vi "Bridge1_Main.vi"(5 "error in (no error)":errorcluster) -> (19 "error out":errorcluster)   [LabVIEW 2020]
doc: "</summary>"
uses:
  CustomersData_class/CustomersData.lvclass
  C:/Projects/DesignPatterns_Trunk/Bridge/DataObject_class/DataObject.lvclass
  Customers_class/Customers.lvclass
panel:
  out "String":string
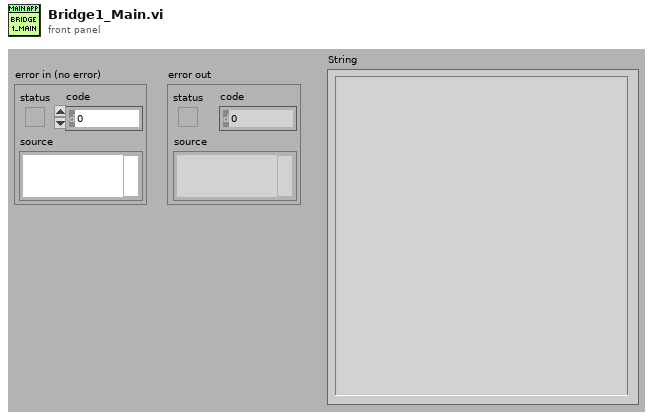
[diagram p1: front panel]
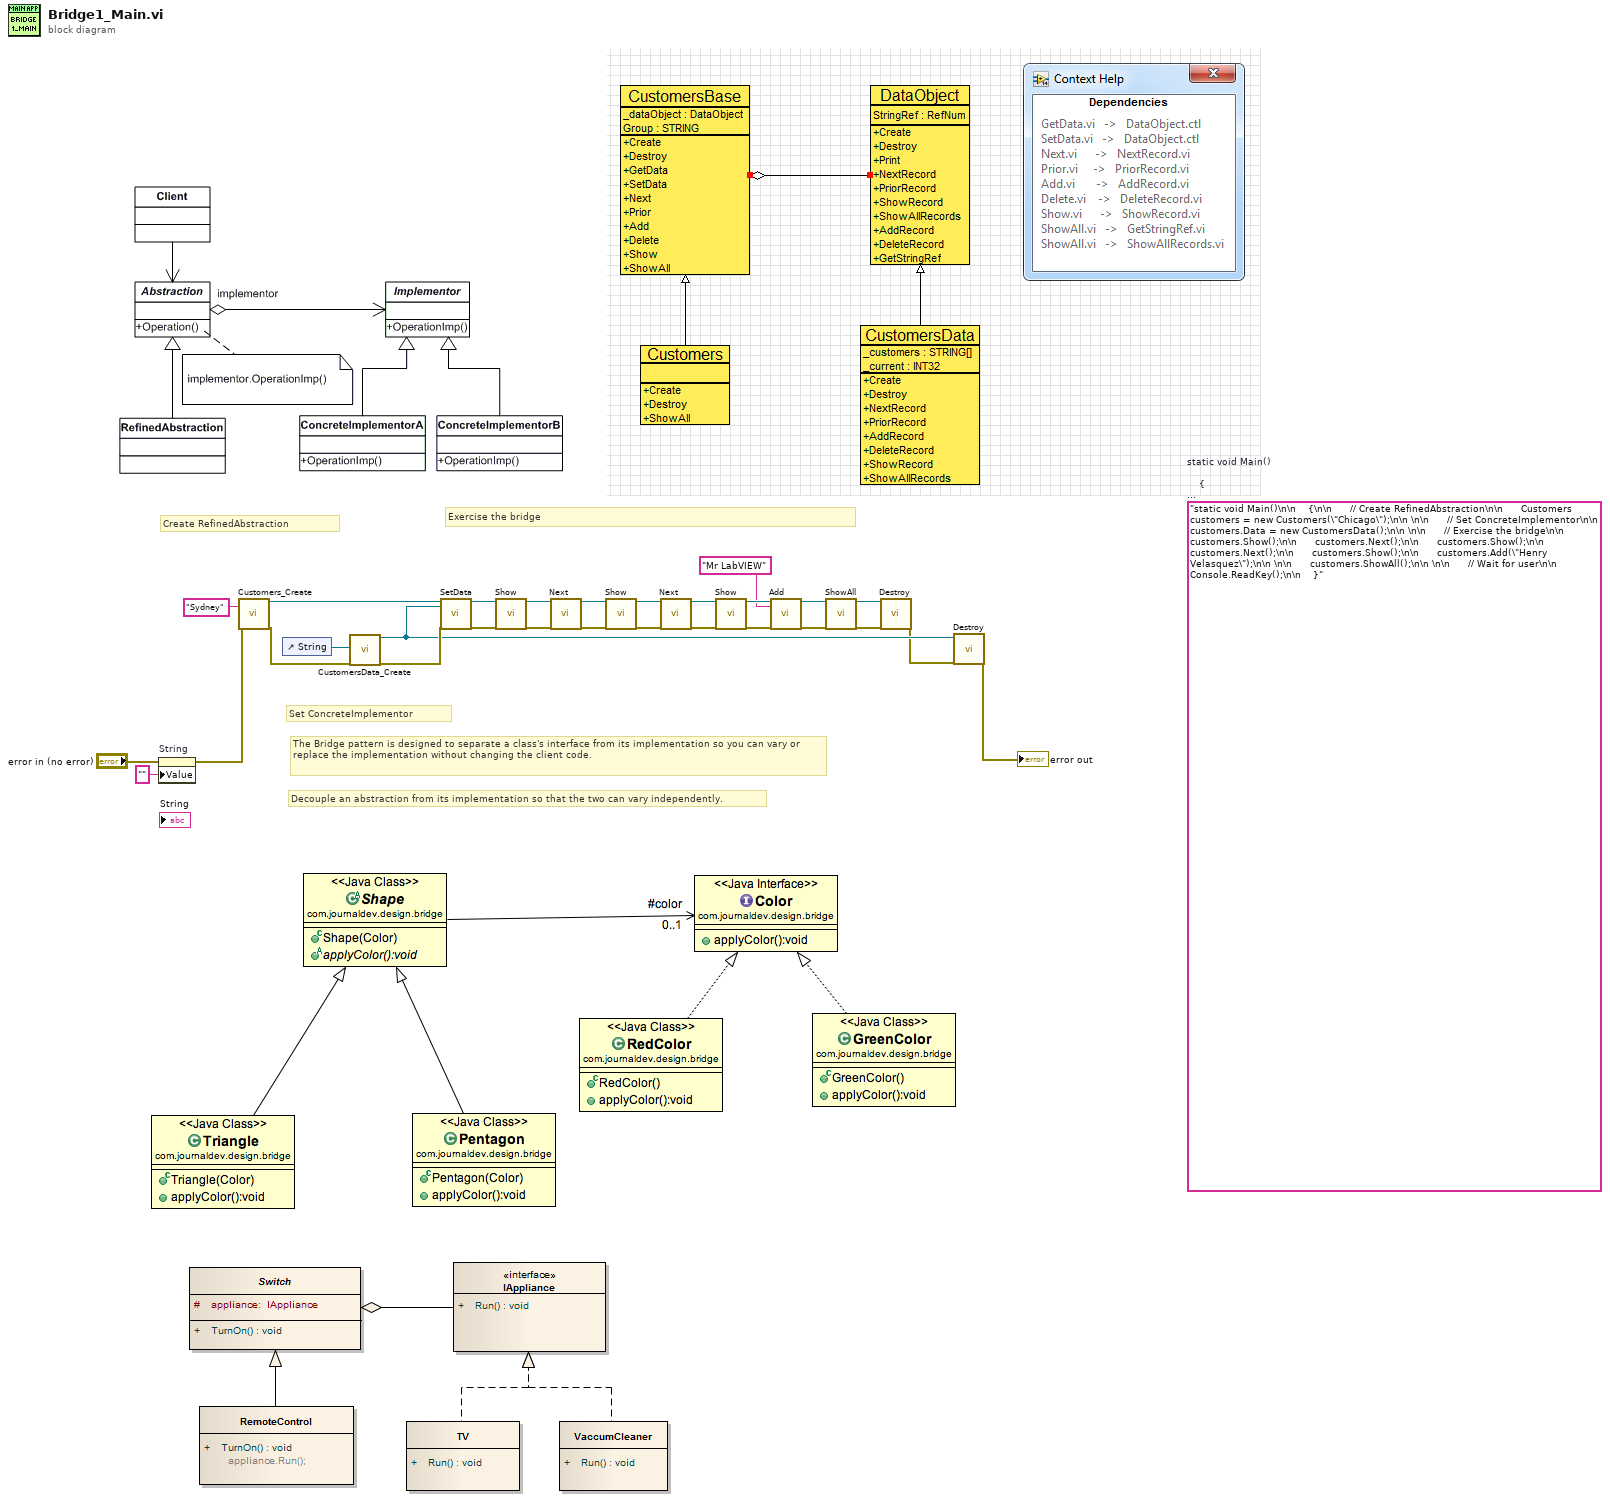
[diagram p0: block diagram]
diagram:
  (unwired) "static void Main()\n\n    {\n\n      // Create RefinedAbstraction\n\n      Customers customers = new Customers(\"Chicago\");\n\n \n\n      // Set ConcreteImplementor\n\n      customers.Data = new CustomersData();\n\n \n\n      // Exercise the bridge\n\n      customers.Show();\n\n      customers.Next();\n\n      customers.Show();\n\n      customers.Next();\n\n      customers.Show();\n\n      customers.Add(\"Henry Velasquez\");\n\n \n\n      customers.ShowAll();\n\n \n\n      // Wait for user\n\n      Console.ReadKey();\n\n    }"  # static void Main()      {        // Create RefinedAbstraction        Customers customers = new Customers("Chicago");           // Set ConcreteImplementor        customers.Data = new CustomersData();           // Exercise the bridge        customers.Show();        customers.Next();        customers.Show();        customers.Next();        customers.Show();        customers.Add("Henry Velasquez");           customers.ShowAll();           // Wait for user        Console.ReadKey();      }
  # "Decouple an abstraction from its implementation so that the two can vary independently."
  # "The Bridge pattern is designed to separate a class's interface from its implementation so you can vary or replace the implementation without changing the client code."
  # "Exercise the bridge"
  # "Set ConcreteImplementor"
  # "Create RefinedAbstraction"
  n1 = property on="String" class="Str"(error in="error in (no error)", "Value"="" ("String")) -> (error out=w2:errorcluster)  [unwired: 1 in, 1 out]
  n2 = call "Customers_Create.vi"("Group"="Sydney", "error in (no error)"=w2) -> ("reference out"=w27:refnum<class "Customers.lvclass">, "error out"=w26:errorcluster)  [unwired: 16 in]
  n3 = control-ref of="String"() -> (w4:refnum<vi>)
  n4 = call "CustomersData_Create.vi"("StringRef"=w4, "error in (no error)"=w26) -> ("reference out"=w7:refnum<class "CustomersData.lvclass">, "error out"=w25:errorcluster)  [unwired: 16 in]
  n5 = call-dynamic "SetData.vi"("reference in"=w27, "Data"=w7, "error in (no error)"=w25) -> ("reference out"=w23:refnum<class "Customers.lvclass">, "error out"=w24:errorcluster)  [unwired: 15 in]
  n6 = call-dynamic "Show.vi"("reference in"=w23, "error in (no error)"=w24) -> ("reference out"=w21:refnum<class "Customers.lvclass">, "error out"=w22:errorcluster)  [unwired: 16 in]
  n7 = call-dynamic "Next.vi"("reference in"=w21, "error in (no error)"=w22) -> ("reference out"=w18:refnum<class "Customers.lvclass">, "error out"=w17:errorcluster)  [unwired: 16 in]
  n8 = call-dynamic "Show.vi"("reference in"=w18, "error in (no error)"=w17) -> ("reference out"=w20:refnum<class "Customers.lvclass">, "error out"=w19:errorcluster)  [unwired: 16 in]
  n9 = call-dynamic "Next.vi"("reference in"=w20, "error in (no error)"=w19) -> ("reference out"=w16:refnum<class "Customers.lvclass">, "error out"=w15:errorcluster)  [unwired: 16 in]
  n10 = call-dynamic "Show.vi"("reference in"=w16, "error in (no error)"=w15) -> ("reference out"=w13:refnum<class "Customers.lvclass">, "error out"=w14:errorcluster)  [unwired: 16 in]
  n11 = call-dynamic "Add.vi"("reference in"=w13, "Customer"="Mr LabVIEW" ("Group"), "error in (no error)"=w14) -> ("reference out"=w11:refnum<class "Customers.lvclass">, "error out"=w10:errorcluster)  [unwired: 15 in]
  n12 = call-dynamic "ShowAll.vi"("reference in"=w11, "error in (no error)"=w10) -> ("reference out"=w8:refnum<class "Customers.lvclass">, "error out"=w9:errorcluster)  [unwired: 16 in]
  n13 = call-dynamic "Destroy.vi"("reference in"=w8, "error in (no error)"=w9) -> ("error out"=w6:errorcluster)  [unwired: 16 in, 1 out]
  n14 = call-dynamic "Destroy.vi"("reference in"=w7, "error in (no error)"=w6) -> ("error out"=→"error out":errorcluster)  [unwired: 16 in, 1 out]
